vi "Add Error.vi"(8 "error in (no error)":errorcluster, 9 "String to Append":string, 11 "Insert Error":bool=TRUE) -> (0 "error out":errorcluster)   [LabVIEW 2021, in "CIF_NIChn_Fifo_Power_DVR.lvclass"]
uses:
  CIF_NIChn_Fifo_Power_DVR.lvclass
  <vilib>/CIF Foundation/CIF Utilities/Errors/Errors_CIF_U.lvlib
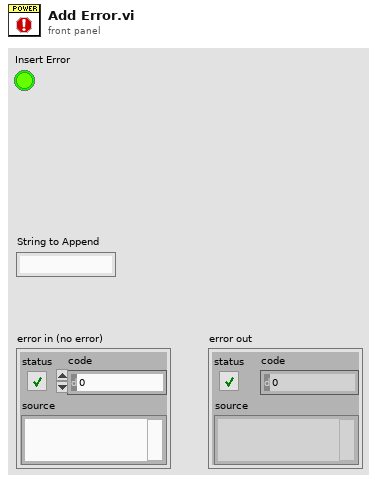
[diagram p1: front panel]
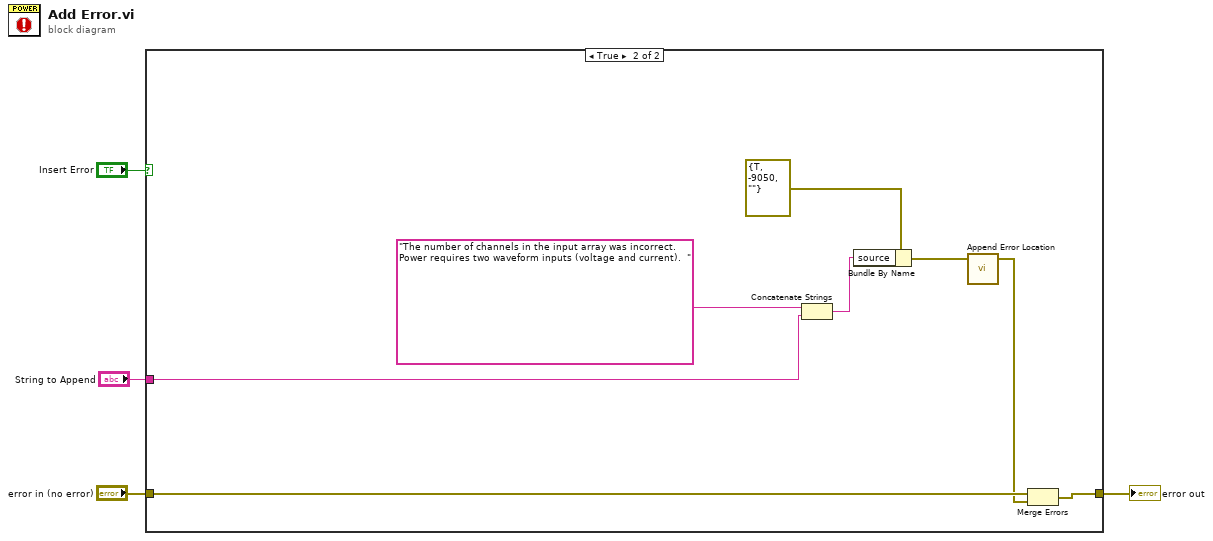
[diagram p0: block diagram]
diagram:
  n1 = case shown="True" "Insert Error" {
    tunnel: [w5 w11] -> w3
    tunnel: "error in (no error)" -> [w5 w12]
    tunnel: "String to Append" -> [_ w13]
    frame False {
    }
    frame True {
      n2 = Concatenate Strings("The number of channels in the input array was incorrect.  Power requires two waveform inputs (voltage and current).  " ("source"), w13) -> (w9:string)
      n3 = Bundle By Name(cluster=errorcluster {"status"=TRUE, "code"=-9050, "source"=""} ("Invalid ID"), "source"=w9) -> (w7:errorcluster)
      n4 = call <vilib>:"Append Error Location.vi"("error in (no error)"=w7) -> ("error out"=w6:errorcluster)  [unwired: 4 in]
      n5 = Merge Errors(w12, w6) -> (w11:errorcluster)
    }
  }
  "error out" <- w3
